vi "RunAutoFile.vi"(8 "error in (no error)":errorcluster, 10 "AutoFile":string) -> (0 "error out":errorcluster)   [LabVIEW 2017]
uses:
  Support/FileCreator/AutoFileDataType.ctl
  Dawgma Programming Library/Controls/PurePursuit/PathFileData.ctl
  Dawgma Programming Library/Controls/PurePursuit/RobotNeededPathData.ctl
  3d26def5-81a8-4255-8638-d6ef2956fa58.vi
  c1318c1c-c8b5-49a0-bd4c-73e64b389bf5.vi
  666bf1a3-f011-47a5-a145-20030bedcc77.vi
  Configuration/Constants.vi
panel:
  out "Auto":T1
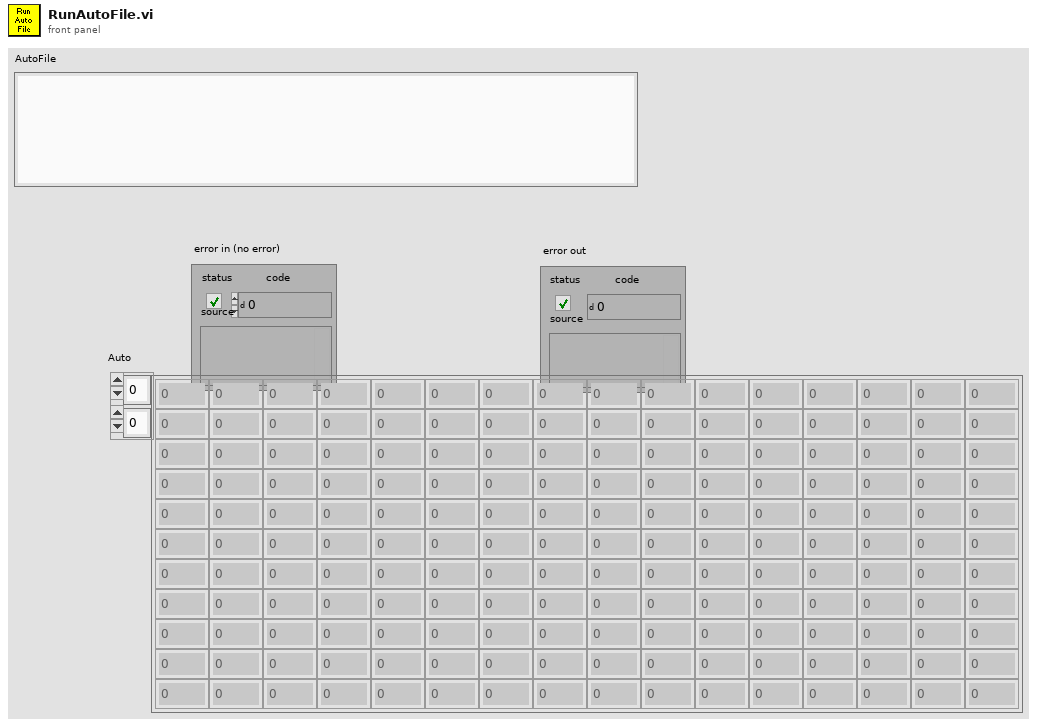
[diagram p1: front panel]
types:
  T1 = typedef "AutoFileDataType.ctl" = dbl[][]
  T2 = typedef "Command Status Info.ctl" = cluster{"Name":string, "Status":T3, "notifier out":T4}
  T3 = typedef "Completion Status.ctl" = enum16{"Successful", "Aborted", "Incomplete"}
  T4 = typedef "Completion Notifier.ctl" = refnum<notifier>
  T5 = typedef "PathFileData.ctl" = cluster{"RobotNeeded":T6, "Meta":cluster{"Path (px)":cluster{i32, i32}[], "RobotWidth":dbl, "RobotLength":dbl, "CenterOfRotYOffset":dbl, "Roundedness":dbl, "StartingPositionPreset":u32, "PathName":string}}
  T6 = typedef "RobotNeededPathData.ctl" = cluster{"Path":cluster{dbl, dbl}[], "MaxVel":dbl, "MaxAccel":dbl, "Backwards?":bool, "PointSpacing":dbl, "LookaheadDist":dbl, "Speed/Curve":dbl, "SlowDistanceAtEnd":dbl, "SlowSpeed":dbl, "MaxDeAccel":dbl}
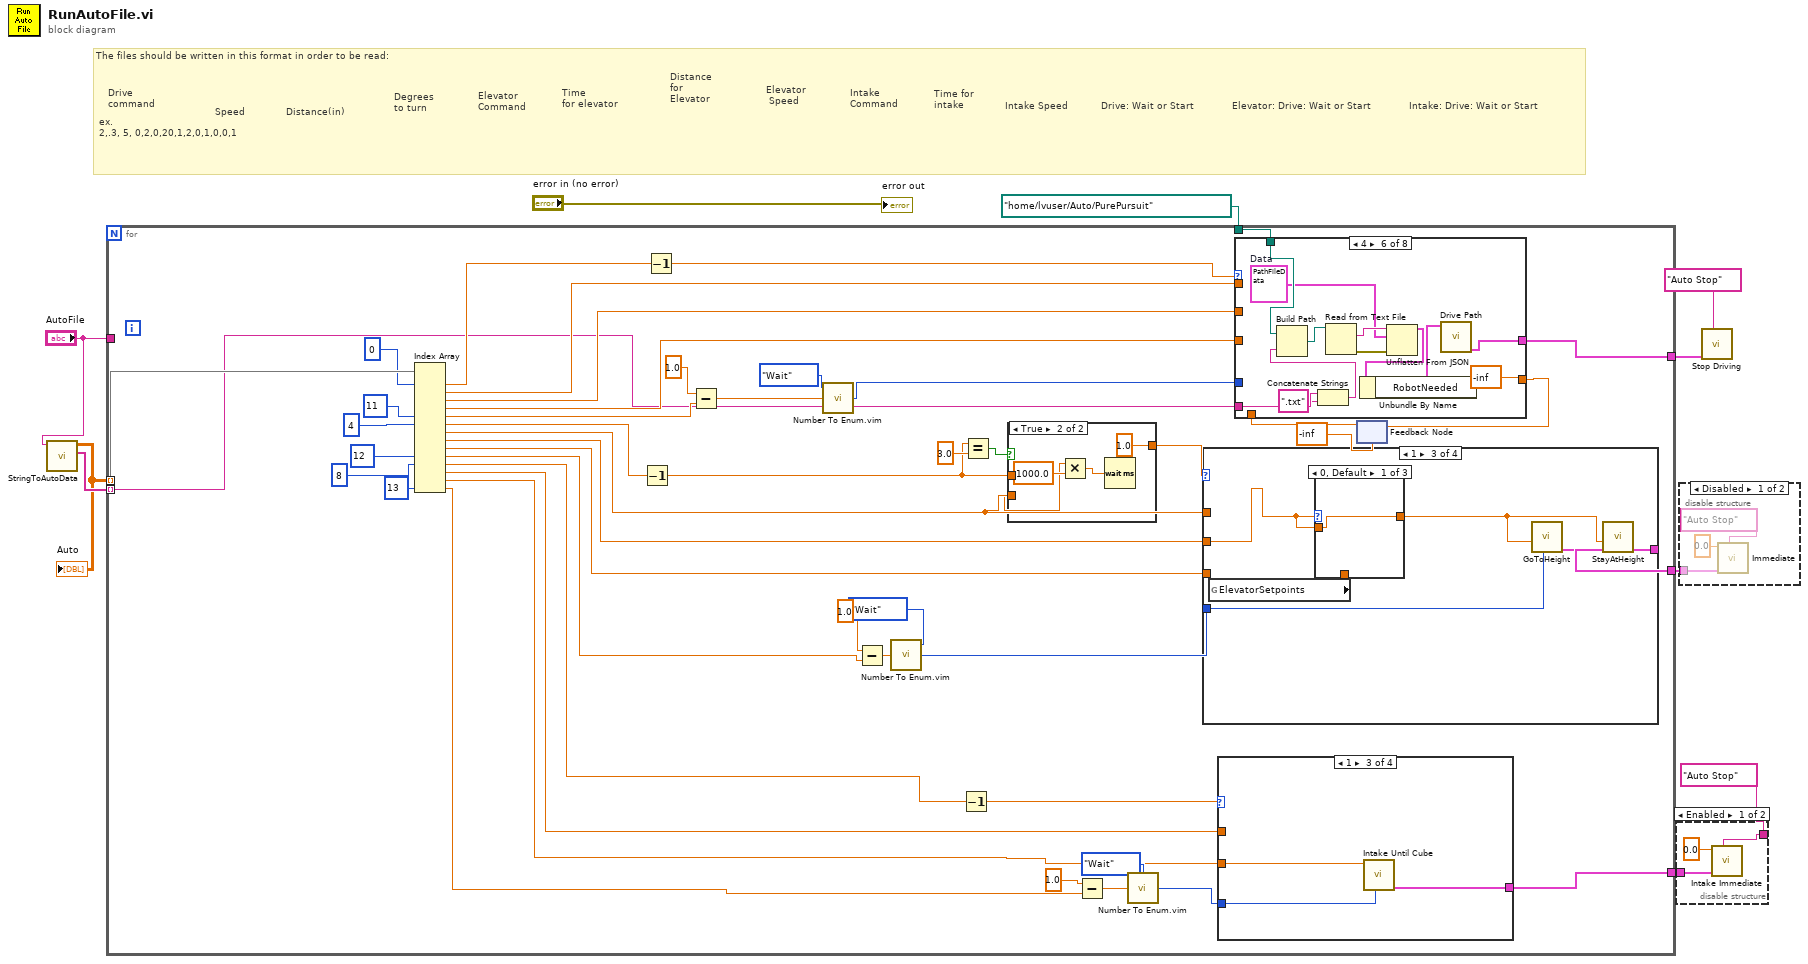
[diagram p0: block diagram]
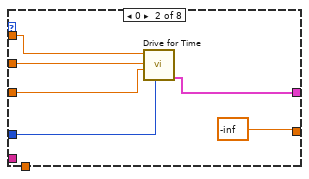
[diagram p5: hidden frame]
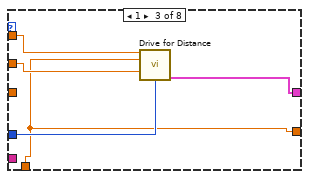
[diagram p6: hidden frame]
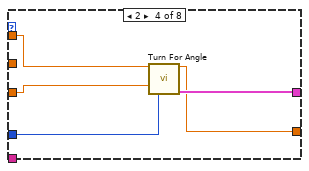
[diagram p7: hidden frame]
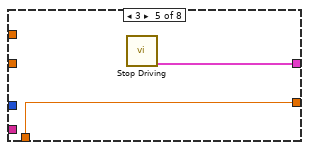
[diagram p8: hidden frame]
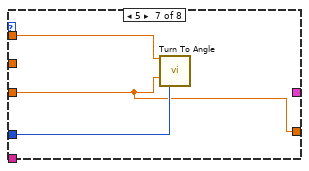
[diagram p9: hidden frame]
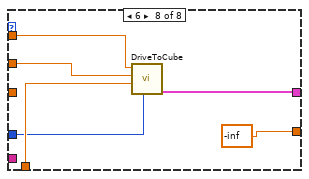
[diagram p10: hidden frame]
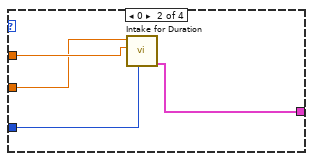
[diagram p12: hidden frame]
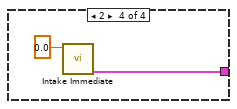
[diagram p13: hidden frame]
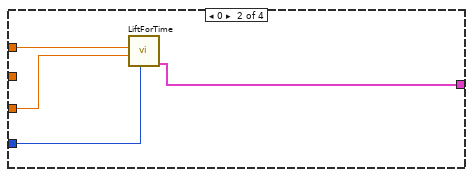
[diagram p15: hidden frame]
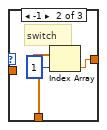
[diagram p16: hidden frame]
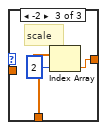
[diagram p17: hidden frame]
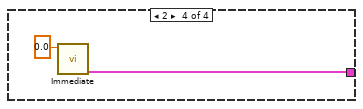
[diagram p18: hidden frame]
diagram:
  # "Intake: Drive: Wait or Start"
  # "Elevator: Drive: Wait or Start"
  # "Drive: Wait or Start"
  # "Time\nfor elevator"
  # "Intake Speed"
  # "Time for \nintake"
  # "Intake \nCommand"
  # "Elevator\n Speed"
  # "Elevator\nCommand"
  # "Distance \nfor\nElevator"
  # "Drive\ncommand"
  # "Degrees \nto turn"
  # "Distance(in)"
  # "Speed"
  # "The files should be written in this format in order to be read:\n                                                                                                                                                                                                                                                                            \n\n\n\n\n ex. \n 2,.3, 5, 0,2,0,20,1,2,0,1,0,0,1"
  n1 = call "StringToAutoData.vi"("String"="AutoFile") -> ("Path File Names"=w4:string[], "Auto"=w3:T1)  [unwired: 9 in]
  "Auto" <- w3
  n2 = for {
    tunnel: "AutoFile" -> [_]
    tunnel: [w55] -> w9
    tunnel: [w54] -> w10
    tunnel: w3 -> [w44] mode=indexing
    tunnel: [w30] -> w6
    tunnel: path "/home/lvuser/Auto/PurePursuit" ("base path") -> [w21]
    tunnel: w4 -> [w20] mode=indexing
    n3 = Index Array(array=w44, index #1=0 ("index"), index #5=11 ("index"), index #6=4 ("index"), index #10=12 ("index"), index #11=8 ("index"), index #14=13 ("index")) -> (element #1=w43:dbl, element #2=w42:dbl, element #3=w41:dbl, element #4=w40:dbl, element #5=w39:dbl, element #6=w38:dbl, element #7=w16:dbl, element #8=w37:dbl, element #9=w36:dbl, element #10=w35:dbl, element #11=w34:dbl, element #12=w33:dbl, element #13=w32:dbl, element #14=w31:dbl)  [unwired: 8 in]
    n4 = Decrement(x=w38) -> (x-1=w14:dbl)
    n5 = Decrement(x=w43) -> (x-1=w57:dbl)
    n6 = Subtract(x=1.0, y=w39) -> (x-y=w51:dbl)
    n7 = call "Number To Enum.vim"("number"=w51, "enum type"=enum16{"Start", "Wait"}."Wait" ("Synchronization")) -> ("number as enum"=w19:enum16{"Start", "Wait"})
    n8 = Subtract(x=1.0, y=w35) -> (x-y=w50:dbl)
    n9 = call "Number To Enum.vim"("number"=w50, "enum type"=enum16{"Start", "Wait"}."Wait" ("Synchronization")) -> ("number as enum"=w23:enum16{"Start", "Wait"})
    n10 = Decrement(x=w34) -> (x-1=w56:dbl)
    n11 = Equal?(x=w14, y=3.0) -> (x = y?=w17:bool)
    n12 = case shown="True" w17 {
      tunnel: w16 -> [_ w61]
      tunnel: [w58 1.0 ("y")] -> w15
      tunnel: w14 -> [w58 _]
      frame False {
      }
      frame True {
        n13 = Multiply(x=w61, y=1000.0) -> (x*y=w60:dbl)
        n14 = Wait (ms)(milliseconds to wait=w60) -> ()  [unwired: 1 out]
      }
    }
    n15 = Subtract(x=1.0, y=w31) -> (x-y=w46:dbl)
    n16 = call "Number To Enum.vim"("number"=w46, "enum type"=enum16{"Start", "Wait"}."Wait" ("Synchronization")) -> ("number as enum"=w22:enum16{"Start", "Wait"})
    n17 = case shown="1" w15 {
      tunnel: w16 -> [_ w115 _ _]
      tunnel: w37 -> [_ _ w117 _]
      tunnel: w36 -> [_ w114 _ _]
      tunnel: [_ w113 w120 w129] -> w54
      tunnel: w23 -> [_ w112 w119 _]
      frame -1, Default {
      }
      frame 0 {
        n18 = call "LiftForTime.vi"("Synchronization"=w112, "Setpoint"=w114, "Duration (s)"=w115) -> ("Command Info Out"=w113:T2)  [unwired: 8 in]
      }
      frame 1 {
        n19 = global read "Constants.vi" "ElevatorSetpoints"() -> (w118:dbl[])
        n20 = case shown="0, Default" w117 {
          tunnel: w118 -> [_ w125 w128]
          tunnel: [w122 w123 w126] -> w116
          tunnel: w117 -> [w122 _ _]
          frame 0, Default {
          }
          frame -1 {
            # "switch"
            n21 = Index Array(array=w125, index=1) -> (element=w123:dbl)
          }
          frame -2 {
            # "scale"
            n22 = Index Array(array=w128, index=2) -> (element=w126:dbl)
          }
        }
        n23 = call "GoToHeight.vi"("Synchronization"=w119, "Setpoint"=w116) -> ("Command Info Out"=w121:T2)  [unwired: 9 in]
        n24 = call "StayAtHeight.vi"("Command Info In"=w121, "Setpoint"=w116) -> ("Command Info Out"=w120:T2)  [unwired: 9 in]
      }
      frame 2 {
        n25 = call "Immediate.vi"("Setpoint"=0.0) -> ("Command Info Out"=w129:T2)  [unwired: 10 in]
      }
    }
    n26 = case shown="1" w56 {
      tunnel: w33 -> [_ w106 _ _]
      tunnel: w32 -> [_ w105 w109 _]
      tunnel: [_ w104 w108 w110] -> w30
      tunnel: w22 -> [_ w103 w107 _]
      frame -1, Default {
      }
      frame 0 {
        n27 = call "Intake for Duration.vi"("Synchronization"=w103, "Duration (s)"=w106, "Speed"=w105) -> ("Command Info Out"=w104:T2)  [unwired: 8 in]
      }
      frame 1 {
        n28 = call "Intake Until Cube.vi"("Synchronization"=w107, "Speed"=w109) -> ("Command Info Out"=w108:T2)  [unwired: 9 in]
      }
      frame 2 {
        n29 = call "Intake Immediate.vi"("Speed"=0.0 ("Setpoint")) -> ("Command Info Out"=w110:T2)  [unwired: 10 in]
      }
    }
    n30 = feedback #1(-inf ("y")) -> (w12:dbl)
    n31 = case shown="4" w57 {
      tunnel: w42 -> [_ w69 w74 w79 _ _ w96 w102]
      tunnel: w41 -> [_ w68 w73 _ _ _ _ w101]
      tunnel: w40 -> [_ w67 _ w78 _ _ w94 _]
      tunnel: [_ w66 w72 w77 w81 w93 _ w98] -> w55
      tunnel: w19 -> [_ w65 w71 w76 _ _ w95 w97]
      tunnel: w20 -> [_ _ _ _ _ w86 _ _]
      tunnel: w21 -> [_ _ _ _ _ w84 _ _]
      tunnel: w12 -> [w63 _ w70 _ w80 _ _ w100]
      tunnel: [w63 -inf ("y") w70 w75 w80 -inf ("y") w94 -inf ("y")] -> w11
      frame -1, Default {
      }
      frame 0 {
        n32 = call "Drive for Time.vi"("Synchronization"=w65, "Seconds"=w67, "Right Speed"=w68, "Left Speed"=w69) -> ("Command Info Out"=w66:T2)  [unwired: 6 in, 1 out]
      }
      frame 1 {
        n33 = call "Drive for Distance.vi"("Speed"=w74, "StartAngle"=w70, "Distance (inch)"=w73, "Synchronication"=w71) -> ("Command Info Out"=w72:T2)  [unwired: 11 in]
      }
      frame 2 {
        n34 = call "Turn For Angle.vi"("Speed"=w79, "Target Angle"=w78, "Synchronication"=w76) -> ("End Angle"=w75:dbl, "Command Info Out"=w77:T2)  [unwired: 11 in]
      }
      frame 3 {
        n35 = call "Stop Driving.vi"() -> ("Command Info Out"=w81:T2)  [unwired: 11 in]
      }
      frame 4 {
        w83 = T5 {"RobotNeeded"={"Path"=[], "MaxVel"=0.0, "MaxAccel"=0.0, "Backwards?"=FALSE, "PointSpacing"=0.0, "LookaheadDist"=0.0, "Speed/Curve"=1.8, "SlowDistanceAtEnd"=12.0, "SlowSpeed"=15.0, "MaxDeAccel"=0.0}, "Meta"={"Path (px)"=[], "RobotWidth"=0.0, "RobotLength"=0.0, "CenterOfRotYOffset"=0.0, "Roundedness"=0.0, "StartingPositionPreset"=0, "PathName"=""}}  # Data
        n36 = Concatenate Strings(w86, ".txt" ("string")) -> (w87:string)
        n37 = Build Path(base path=w84, name or relative path=w87) -> (appended path=w88:path)
        n38 = Read from Text File(file (use dialog)=w88) -> (text=w89:string, error out=w90:errorcluster)  [unwired: 3 in, 2 out]
        n39 = Unflatten From JSON(JSON string=w89, type and defaults=w83, error in (no error)=w90) -> (value=w91:T5)  [unwired: 4 in, 1 out]
        n40 = Unbundle By Name(w91) -> ("RobotNeeded"=w92:T6)
        n41 = call "Drive Path.vi"("Path"=w92) -> ("Command Info Out"=w93:T2)  [unwired: 10 in]
      }
      frame 5 {
        n42 = call "Turn To Angle.vi"("Speed"=w96, "Target Angle"=w94, "Synchronication"=w95) -> ()  [unwired: 12 in, 1 out]
      }
      frame 6 {
        n43 = call "DriveToCube.vi"("Synchronication"=w97, "StartAngle"=w100, "Distance"=w101, "Speed"=w102) -> ("Command Info Out"=w98:T2)  [unwired: 7 in]
      }
    }
    n44 = feedback-in #1(w11) -> ()
  }
  n45 = disable-structure shown="Enabled" {
    disable-tunnel: w6 -> [w132 _]
    disable-tunnel: "Auto Stop" ("Description") -> [w131 _]
    frame Enabled {
      n46 = call "Intake Immediate.vi"("Description"=w131, "Command Info In"=w132, "Speed"=0.0 ("Setpoint")) -> ()  [unwired: 8 in, 1 out]
    }
    frame Disabled {
    }
  }
  n47 = disable-structure shown="Disabled" {
    disable-tunnel: w10 -> [w135 _]
    frame Disabled {
      n48 = call "Immediate.vi"("Description"="Auto Stop", "Command Info In"=w135, "Setpoint"=0.0) -> ()  [unwired: 8 in, 1 out]
    }
    frame Enabled {
    }
  }
  n49 = call "Stop Driving.vi"("Description"="Auto Stop", "Command Info In"=w9) -> ()  [unwired: 9 in, 1 out]
  "error out" <- "error in (no error)"
